vi "Ejemplo4_operaciones_Numericas.vi"() -> ()   [LabVIEW 2020]
panel:
  out "Resultado Division":dbl
  out "Resultado Multiplicacion":u16
  out "Resultado Resta":u8
  out "Resultado Suma":u8
  in  "Numero 5":dbl(slide) scale=0.0..100.0
  in  "Numero 4":u8(slide) scale=0.0..100.0
  in  "Numero 3":u8(slide) scale=0.0..100.0
  in  "Numero 2":u8(slide) scale=0.0..100.0
  in  "Numero 1":u8(slide) scale=0.0..100.0
  # "Operaciones Numericas"
  # "70"
  # "30"
  # "250"
  # "5"
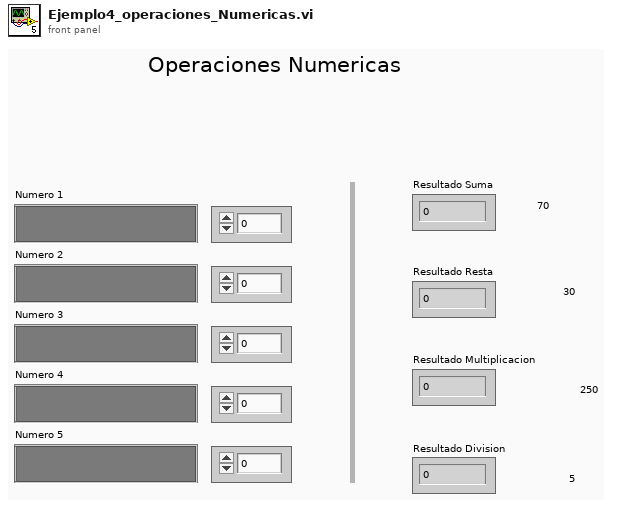
[diagram p1: front panel]
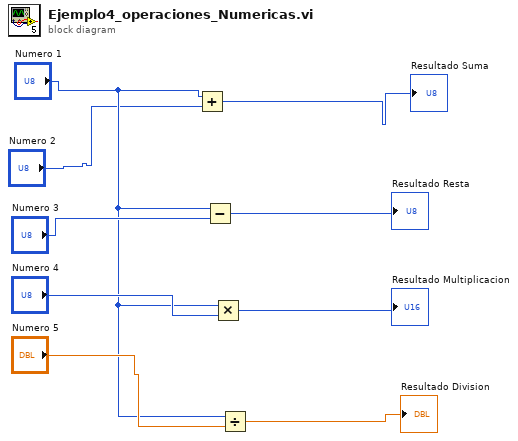
[diagram p0: block diagram]
diagram:
  n1 = Add(x="Numero 1", y="Numero 2") -> (x+y=→"Resultado Suma":u8)
  n2 = Subtract(x="Numero 1", y="Numero 3") -> (x-y=→"Resultado Resta":u8)
  n3 = Multiply(x="Numero 1", y="Numero 4") -> (x*y=→"Resultado Multiplicacion":u8)
  n4 = Divide(x="Numero 1", y="Numero 5") -> (x/y=→"Resultado Division":dbl)
